vi "Invert_1D_Array.vi"(6 "Invert?":bool, 9 "Array IN":dbl[](array[numeric])) -> (1 "Array OUT":dbl[](array[numeric]))   [LabVIEW 2018]
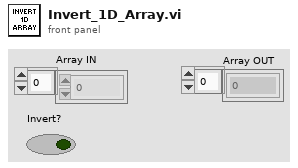
[diagram p1: front panel]
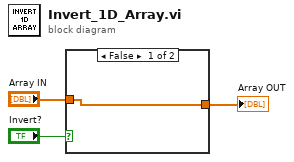
[diagram p0: block diagram]
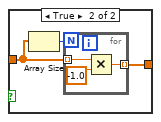
[diagram p2: hidden frame]
diagram:
  n1 = case shown="False" "Invert?" {
    tunnel: "Array IN" -> [w4 w6]
    tunnel: [w4 w5] -> w2
    frame False {
    }
    frame True {
      n2 = Array Size(array=w6) -> (size(s)=w7:i32)
      n3 = for {
        N: w7 -> [_]
        tunnel: w6 -> [w10] mode=indexing
        tunnel: [w8] -> w5 mode=indexing
        n4 = Multiply(x=w10, y=-1.0) -> (x*y=w8:dbl)
      }
    }
  }
  "Array OUT" <- w2
